vi "MCCMSG Set Slow Current Inj Enable.vi"(8 "error in (no error)":errorcluster, 9 "pnError":i32, 10 "bEnable":i32, 11 "hMCCmsg":i32) -> (0 "error out":errorcluster, 1 "pnError out":i32, 3 "function return":i32)   [LabVIEW 2012, in "MultiClamp 700B Controls.lvlib" / "AxMultiClampMsg.lvlib"]
doc: "AXMCCMSG BOOL WINAPI MCCMSG_SetSlowCurrentInjEnable(HMCCMSG hMCCmsg, BOOL bEnable, int *pnError);"
uses:
  AxMultiClampMsg.lvlib
  AxMultiClampMsg.dll
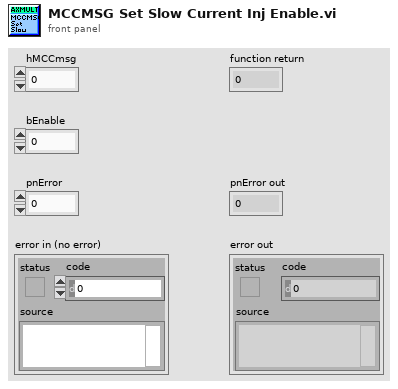
[diagram p1: front panel]
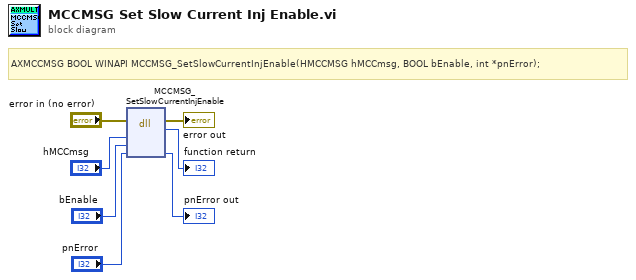
[diagram p0: block diagram]
diagram:
  # "AXMCCMSG BOOL WINAPI MCCMSG_SetSlowCurrentInjEnable(HMCCMSG hMCCmsg, BOOL bEnable, int *pnError);"
  n1 = dll-call lib="C:/Users/LAA12/Desktop/Rita/Multiclamp 700B VIs/AxMultiClampMsg/AxMultiClampMsg.*" fn="MCCMSG_SetSlowCurrentInjEnable"(error in="error in (no error)", "hMCCmsg"="hMCCmsg", "bEnable"="bEnable", "pnError"="pnError") -> (error out=→"error out":errorcluster, →"function return":i32, "pnError"=→"pnError out":i32)  [unwired: 4 in, 1 out]
